vi "GSCS_PDA_Control_GUI.vi"(4 "error in (no error)":errorcluster, 7 "TCP Network Connection Refnum":refnum<k5>) -> (0 "error out":errorcluster)   [LabVIEW 2015]
doc: "Use this template to build a PDA VI for Pocket PC 2002 devices or emulators."
panel:
  out "Status":string
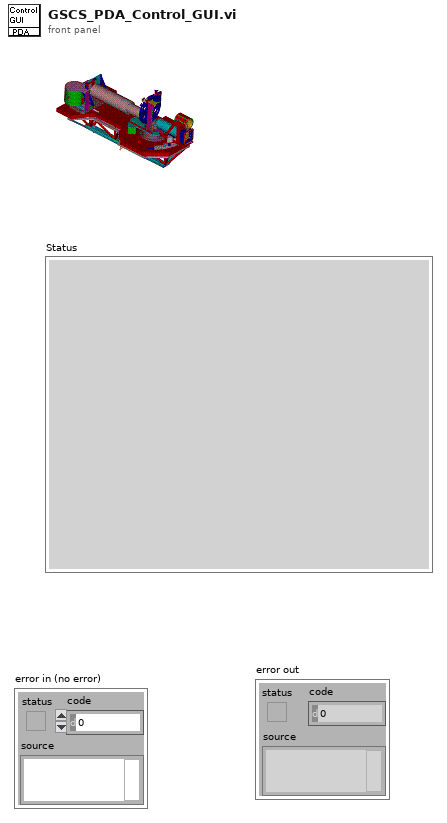
[diagram p1: front panel]
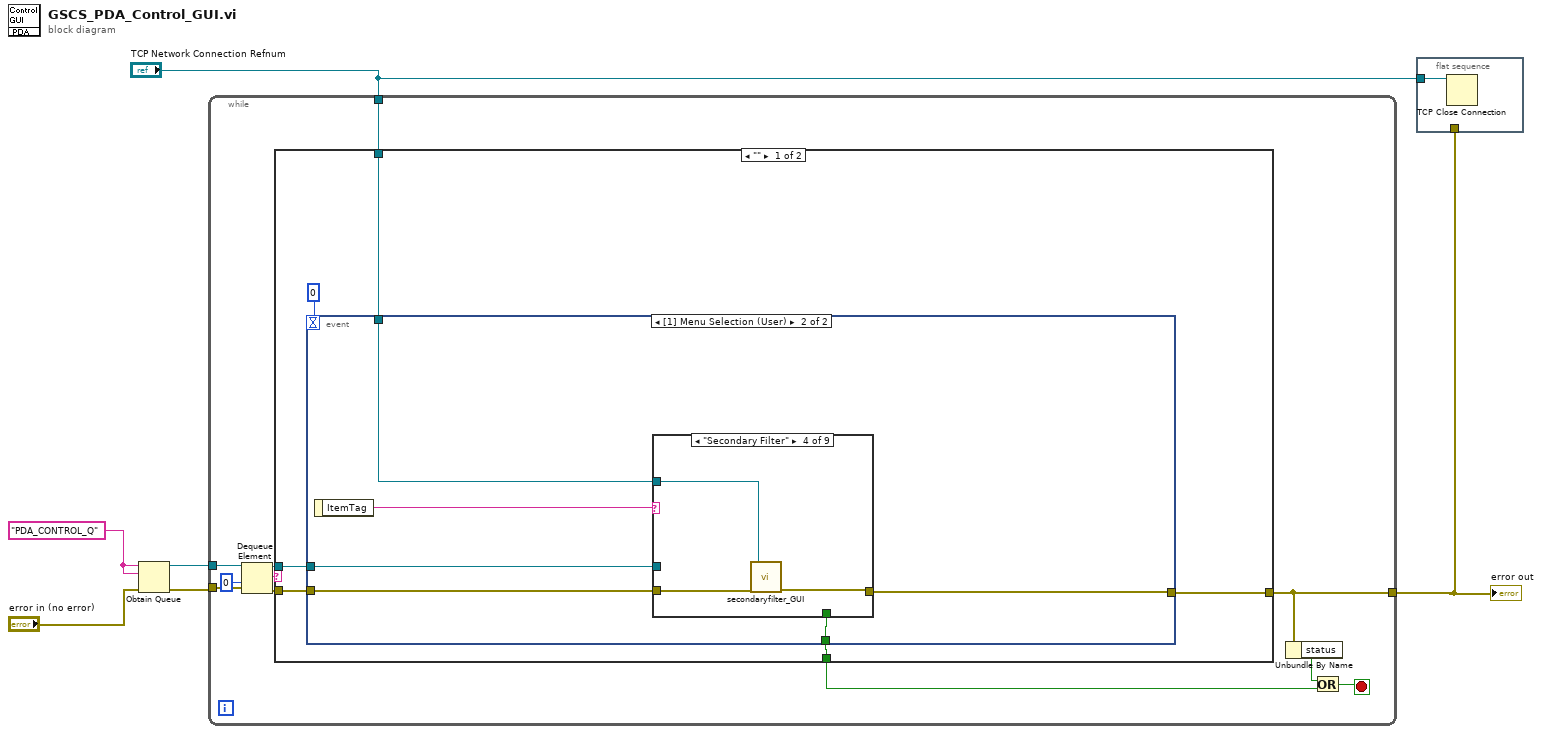
[diagram p0: block diagram]
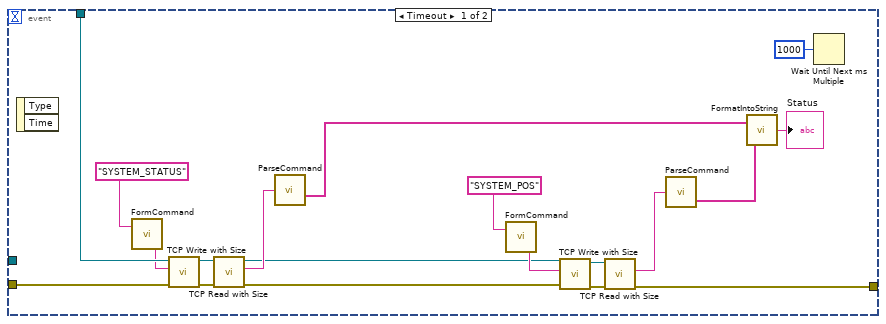
[diagram p2: hidden frame]
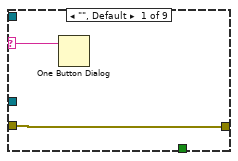
[diagram p3: hidden frame]
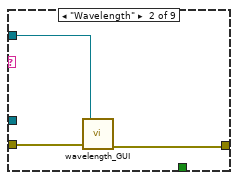
[diagram p4: hidden frame]
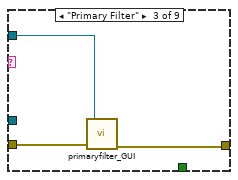
[diagram p5: hidden frame]
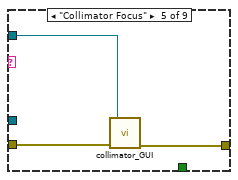
[diagram p6: hidden frame]
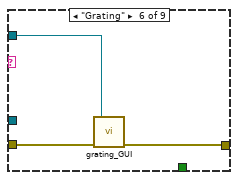
[diagram p7: hidden frame]
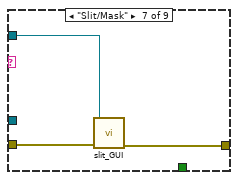
[diagram p8: hidden frame]
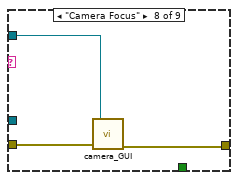
[diagram p9: hidden frame]
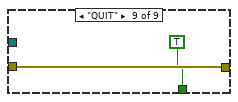
[diagram p10: hidden frame]
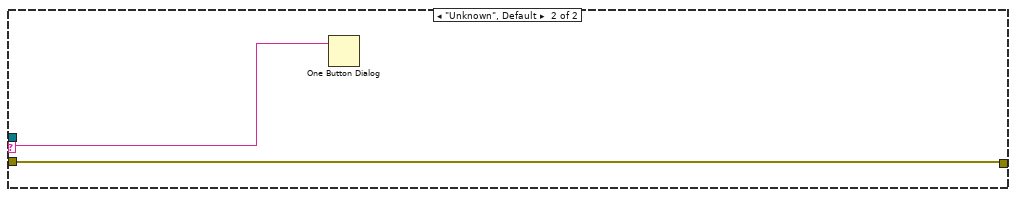
[diagram p11: hidden frame]
diagram:
  w5 = "PDA_CONTROL_Q" ("name (unnamed)")
  n1 = Obtain Queue(name (unnamed)=w5, element data type=w5, error in (no error)="error in (no error)") -> (queue out=w3:refnum<queue>, error out=w4:errorcluster)  [unwired: 2 in, 1 out]
  n2 = while {
    tunnel: w4 -> [w13]
    tunnel: [w15] -> w1
    tunnel: w3 -> [w14]
    tunnel: "TCP Network Connection Refnum" -> [w7]
    stop <- w17 stop-if-true
    n3 = Dequeue Element(queue=w14, timeout in ms (-1)=0, error in (no error)=w13) -> (queue out=w10:refnum<queue>, element=w9:string, error out=w11:errorcluster)  [unwired: 1 out]
    n4 = case shown="\"\"" w9 {
      selector: w9 -> [_ w75]
      tunnel: [w23 w74] -> w15
      tunnel: w11 -> [w22 w74]
      tunnel: w10 -> [w21 _]
      tunnel: [w19 _] -> w8
      tunnel: w7 -> [w18 _]
      frame "" {
        n5 = event shown="[1] Menu Selection (User)" {
          selector: _ -> [_ _]
          dyn-events: _ -> [_ _]
          timeout: 0 -> [_ _]
          tunnel: w22 -> [w39 w47]
          tunnel: [w24 w45] -> w23
          tunnel: w21 -> [_ w46]
          tunnel: [_ w44] -> w19
          tunnel: w18 -> [w38 w43]
          event Timeout {
            n6 = event-data() -> ()  [unwired: 1 in, 2 out]
            n7 = call "FormCommand.vi"("Command"="SYSTEM_STATUS") -> ("Command string"=w35:string)  [unwired: 1 in]
            n8 = call "TCP Write with Size.vi"("error in (no error)"=w39, "data in"=w35, "connection ID"=w38) -> ("error out"=w41:errorcluster, "connection ID out"=w42:refnum<k5>)  [unwired: 6 in, 1 out]
            n9 = call "TCP Read with Size.vi"("error in (no error)"=w41, "connection ID"=w42) -> ("error out"=w28:errorcluster, "data out"=w37:string, "connection ID out"=w29:refnum<k5>)  [unwired: 7 in]
            n10 = call "ParseCommand.vi"("Command string"=w37) -> ("Parameters"=w27:string[])  [unwired: 1 out]
            n11 = call "FormCommand.vi"("Command"="SYSTEM_POS") -> ("Command string"=w30:string)  [unwired: 1 in]
            n12 = call "TCP Write with Size.vi"("error in (no error)"=w28, "data in"=w30, "connection ID"=w29) -> ("error out"=w33:errorcluster, "connection ID out"=w34:refnum<k5>)  [unwired: 6 in, 1 out]
            n13 = call "TCP Read with Size.vi"("error in (no error)"=w33, "connection ID"=w34) -> ("error out"=w24:errorcluster, "data out"=w32:string)  [unwired: 7 in, 1 out]
            n14 = call "ParseCommand.vi"("Command string"=w32) -> ("Parameters"=w26:string[])  [unwired: 1 out]
            n15 = call "FormatIntoString.vi"("System Pos"=w26, "System Status"=w27) -> ("String out"=→"Status":string)
            n16 = Wait Until Next ms Multiple(millisecond multiple=u32 1000 ("milliseconds to wait")) -> ()  [unwired: 1 out]
          }
          event Menu Selection (User) {
            n17 = event-data() -> ("ItemTag"=w48:string)  [unwired: 1 in]
            n18 = case shown="\"Secondary Filter\"" w48 {
              selector: w48 -> [w49 _ _ _ _ _ _ _ _]
              tunnel: w47 -> [w50 w53 w56 w59 w62 w65 w68 w71 w73]
              tunnel: w46 -> [_ _ _ _ _ _ _ _ _]
              tunnel: [w50 w51 w55 w57 w60 w63 w66 w69 w73] -> w45
              tunnel: [_ _ _ _ _ _ _ _ TRUE] -> w44
              tunnel: w43 -> [_ w52 w54 w58 w61 w64 w67 w70 _]
              frame "", Default {
                n19 = One Button Dialog(message=w49) -> ()  [unwired: 1 in, 1 out]
              }
              frame "Wavelength" {
                n20 = call "wavelength_GUI.vi"("error in (no error)"=w53, "connection ID"=w52) -> ("error out"=w51:errorcluster)  [unwired: 5 in]
              }
              frame "Primary Filter" {
                n21 = call "primaryfilter_GUI.vi"("error in (no error)"=w56, "connection ID"=w54) -> ("error out"=w55:errorcluster)  [unwired: 5 in]
              }
              frame "Secondary Filter" {
                n22 = call "secondaryfilter_GUI.vi"("error in (no error)"=w59, "connection ID"=w58) -> ("error out"=w57:errorcluster)  [unwired: 5 in]
              }
              frame "Collimator Focus" {
                n23 = call "collimator_GUI.vi"("error in (no error)"=w62, "connection ID"=w61) -> ("error out"=w60:errorcluster)  [unwired: 5 in]
              }
              frame "Grating" {
                n24 = call "grating_GUI.vi"("error in (no error)"=w65, "connection ID"=w64) -> ("error out"=w63:errorcluster)  [unwired: 5 in]
              }
              frame "Slit/Mask" {
                n25 = call "slit_GUI.vi"("error in (no error)"=w68, "connection ID"=w67) -> ("error out"=w66:errorcluster)  [unwired: 5 in]
              }
              frame "Camera Focus" {
                n26 = call "camera_GUI.vi"("error in (no error)"=w71, "connection ID"=w70) -> ("error out"=w69:errorcluster)  [unwired: 5 in]
              }
              frame "QUIT" {
              }
            }
          }
        }
      }
      frame "Unknown", Default {
        n27 = One Button Dialog(message=w75) -> ()  [unwired: 1 in, 1 out]
      }
    }
    n28 = Unbundle By Name(w15) -> ("status"=w16:bool)
    n29 = Or(x=w16, y=w8) -> (x .or. y?=w17:bool)
  }
  "error out" <- w1
  n30 = flat-sequence {
    tunnel: "TCP Network Connection Refnum" -> [w76]
    tunnel: w1 -> [_]
    frame #0 {
      n31 = TCP Close Connection(connection ID=w76) -> ()  [unwired: 2 in, 2 out]
    }
  }
